vi "FGV_TileVisible.vi"(7 "Tile Visible FGV":T1, 10 "Value":bool, 11 "Index":i16) -> (2 "Value Out":bool)   [LabVIEW 2020]
uses:
  FGV_TileVisibleEnum.ctl
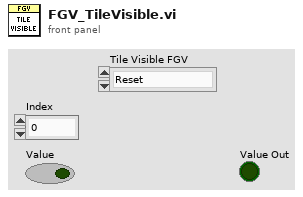
[diagram p1: front panel]
types:
  T1 = typedef "FGV_TileVisibleEnum.ctl" = enum16{"Reset", "Set Value", "Read Value"}
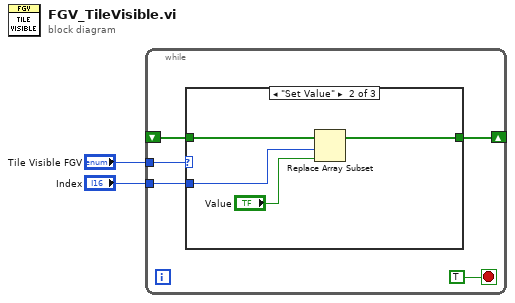
[diagram p0: block diagram]
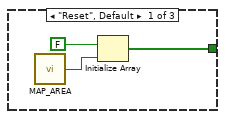
[diagram p2: hidden frame]
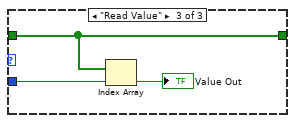
[diagram p3: hidden frame]
diagram:
  n1 = while {
    tunnel: "Tile Visible FGV" -> [w6]
    shift-right: [w5] -> _
    shift-left: _ -> [w4]
    tunnel: "Index" -> [w3]
    stop <- TRUE stop-if-true
    n2 = case shown="\"Set Value\"" w6 {
      tunnel: [w8 w13 w16] -> w5
      tunnel: w4 -> [_ w14 w16]
      tunnel: w3 -> [_ w12 w17]
      frame "Reset", Default {
        n3 = call "MAP_AREA.vi"() -> ("MAP_DIM"=w10:i16)
        n4 = Initialize Array(FALSE, w10) -> (w8:bool[])
      }
      frame "Set Value" {
        n5 = Replace Array Subset(array=w14, new element="Value", index=w12) -> (w13:bool[])
      }
      frame "Read Value" {
        n6 = Index Array(array=w16, index=w17) -> (element=→"Value Out":bool)
      }
    }
  }
